vi "Write Channel 2 U8 Array.vi"(8 "error in (no error)":errorcluster, 10 "Channel 2 U8 Array":u8[](array[numeric]), 11 "Conversion in":refnum<class "Conversion.lvclass">) -> (0 "error out":errorcluster, 3 "Conversion out":refnum<class "Conversion.lvclass">)   [LabVIEW 2023, in "Conversion.lvclass"]
uses:
  Conversion.lvclass
  Conversion.lvclass/Conversion.ctl
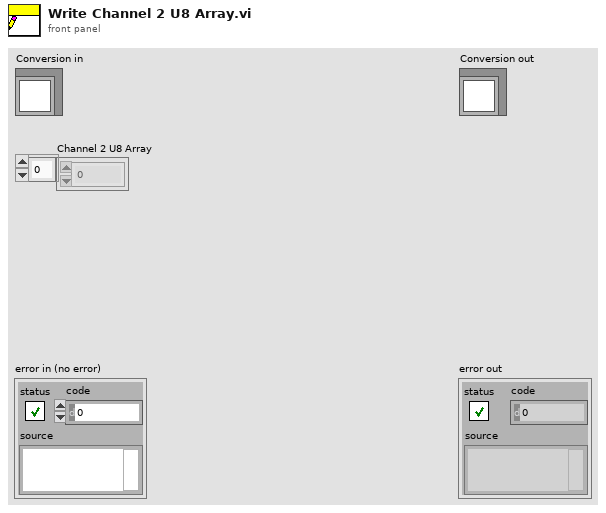
[diagram p1: front panel]
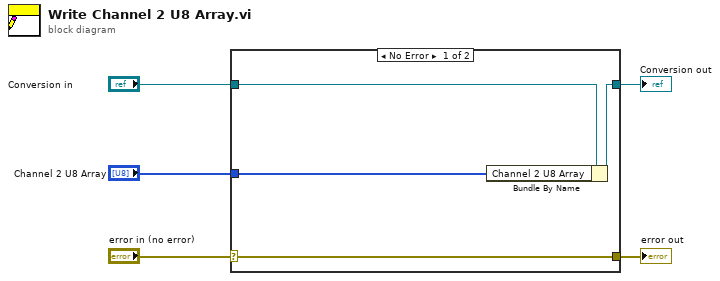
[diagram p0: block diagram]
diagram:
  n1 = case shown="No Error" "error in (no error)" {
    selector: "error in (no error)" -> [w9 w10]
    tunnel: [w9 w10] -> w4
    tunnel: [w7 w11] -> w2
    tunnel: "Conversion in" -> [w8 w11]
    tunnel: "Channel 2 U8 Array" -> [w6 _]
    frame No Error {
      n2 = Bundle By Name(cluster=w8, "Channel 2 U8 Array"=w6) -> (w7:refnum<class "Conversion.lvclass">)
    }
    frame Error {
    }
  }
  "error out" <- w4
  "Conversion out" <- w2
